vi "Assemble QuadViewManager.vi"(0 "Top View":refnum<class "IViewable.lvclass">, 1 "Bottom View":refnum<class "IViewable.lvclass">) -> (7 "QuadViewManager out":refnum<class "TowViewManager.lvclass">)   [LabVIEW 2017, in "TowViewManager.lvlib" / "TowViewManager.lvclass"]
doc: "<License>\nCopyright © 2017 Composed Systems, LLC | All rights reserved\nwww.composed.io\n\nAuthor: Ethan Stern <ethan.stern@composed.io>\n\nThis software is provided \"AS IS\" WITHOUT WARRANTIES, either express or implied, AND IS FOR EDUCATIONAL PURPOSES ONLY.\n</License>"
uses:
  <vilib>/gpm_packages/TestSystem/Views/UpDown ViewManager/TowViewManager.lvclass
  C:/Program Files/National Instruments/LabVIEW 2017/vi.lib/gpm_packages/@cs/mva-viewable/Source/IViewManager/IViewManager/IViewManager.lvclass
  <vilib>/gpm_packages/@cs/mva-viewable/Source/IViewable/IViewable/IViewable.lvclass
  <vilib>/gpm_packages/@cs/mva-viewable/Source/IViewManager/IViewManager Messages/Launch Nested Views Msg/Launch Nested Views Msg.lvclass/Launch Nested Views Msg.ctl
  <vilib>/gpm_packages/@cs/mva-viewable/Source/IViewManager/IViewManager/IViewManager.lvclass/IViewManager.ctl
  <vilib>/gpm_packages/@cs/mva-viewable/Source/IViewManager/IViewManager Messages/Launch Nested Views Msg/Pack Launch Nested Views Msg.vi
  <vilib>/gpm_packages/@cs/mva-viewable/Source/IViewManager/IViewManager Messages/Launch Nested Views Msg/Launch Nested Views Msg.lvclass
  <vilib>/gpm_packages/@cs/mva-viewable/Source/IViewManager/IViewManager/IViewManager.lvclass
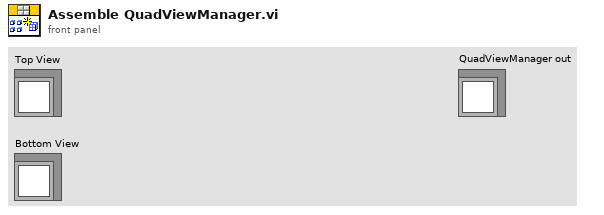
[diagram p1: front panel]
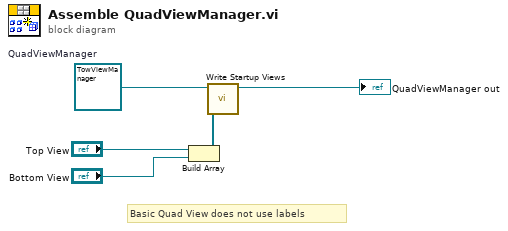
[diagram p0: block diagram]
diagram:
  w5 = refnum<class "TowViewManager.lvclass"> refnum  # QuadViewManager
  # "Basic Quad View does not use labels"
  n1 = Build Array("Top View", "Bottom View") -> (w2:refnum<class "IViewable.lvclass">[])
  n2 = call <vilib>:"Write Startup Views.vi"("Startup Views"=w2, "IViewManager in"=w5) -> ("IViewManager out"=→"QuadViewManager out":refnum<class "TowViewManager.lvclass">)  [unwired: 9 in]
